vi "Intake Arm Controller.vi"(8 "error in":errorcluster) -> ()   [LabVIEW 2020]
doc: "This VI executes continuously carrying out the current operation and responding to updates or new operations. It will often contain the timing or control code that is difficult to place directly in TeleOp. This VI generally opens all sensors and motors and isolates the rest of the robot code from knowing how the operations are carried out."
uses:
  <vilib>/Rock Robotics/WPI/Framework/Completion Status.ctl
  Intake Arm Setpoints.ctl
  Intake Arm Operations.ctl
  <vilib>/Rock Robotics/WPI/Solenoid/WPI_SolenoidValue.ctl
  <vilib>/Rock Robotics/WPI/Solenoid/WPI_SolenoidChannel.ctl
  <vilib>/Rock Robotics/WPI/SafetyOutput/WPI_SafetyOutputConfigMenu.ctl
  <vilib>/Rock Robotics/WPI/Solenoid/WPI_SolenoidOpenDouble.vi
  <vilib>/Rock Robotics/WPI/Solenoid/WPI_SolenoidSetEnum.vi
  <vilib>/Rock Robotics/Network Tables/NT Write Number.vi
panel:
  in  "Interactive Values":T1
  out "Current\nCmd":string
  in  "Buttons":cluster{"Execute Cmd":bool, "Abort Cmd":bool}
  out "Command Timing":cluster{"Start Time (ms)":u32, "Iterations":i32}
  out "Status":T4
  # "Tip: It may be helpful to observe inputs and sensor values.\nYou may also want to display tuning or debugging controls."
  # "Interactive Command: You may fill in the settings for a command\nand schedule it with the Execute button. You can observe and abort\nany command while fine tuning the code for the controller."
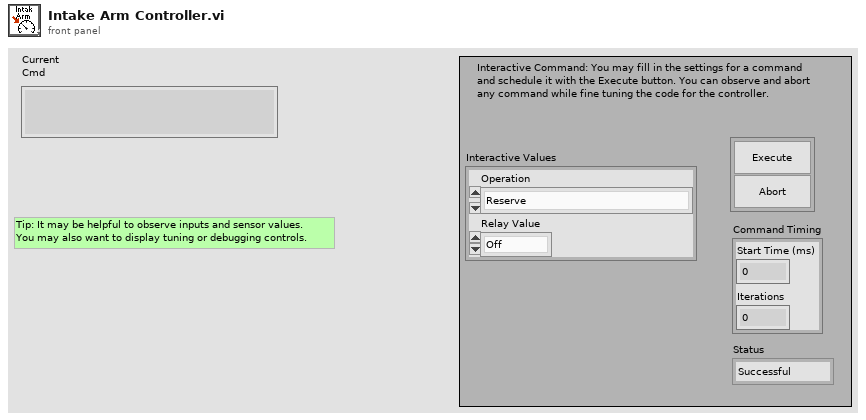
[diagram p1: front panel]
types:
  T1 = typedef "Intake Arm Setpoints.ctl" = cluster{"Operation":T2, "Relay Value":T3}
  T2 = typedef "Intake Arm Operations.ctl" = enum16{"Reserve", "Read Current", "Immediate", "Intake Arm Immediate", "Down", "Up"}
  T3 = typedef "WPI_SolenoidValue.ctl" = enum16{"Off", "On", "Forward", "Reverse"}
  T4 = typedef "Completion Status.ctl" = enum16{"Successful", "Aborted", "Incomplete"}
  T5 = typedef "WPI_SolenoidChannel.ctl" = enum8{"Solenoid 0", "Solenoid 1", "Solenoid 2", "Solenoid 3", "Solenoid 4", "Solenoid 5", "Solenoid 6", "Solenoid 7", "Solenoid 8", "Solenoid 9", "Solenoid 10", "Solenoid 11", "Solenoid 12", "Solenoid 13", "Solenoid 14", "Solenoid 15", "Invalid"}
  T6 = typedef "WPI_SafetyOutputConfigMenu.ctl" = enum16{"Enable", "Disable"}
  T7 = typedef "WPI_SolenoidDevRef.ctl" = cluster{"DevStatus":errorcluster, "Pneumatics Control Module":u8, "Forward Solenoid Channel":T5, "Reverse Solenoid Channel":T5}
  T8 = typedef "Command Status Info.ctl" = cluster{"Name":string, "Status":T4, "notifier out":T9}
  T9 = typedef "Completion Notifier.ctl" = refnum<notifier>
  T10 = cluster{"Current Command":T1, "Command Timing":cluster{"Start Time (ms)":u32, "Iterations":i32}, "Command Arguments":cluster{"Command Info":T8, "Description":string, "Default Command":T1, "queue out":refnum<queue>, "Subsystem Name":string}}
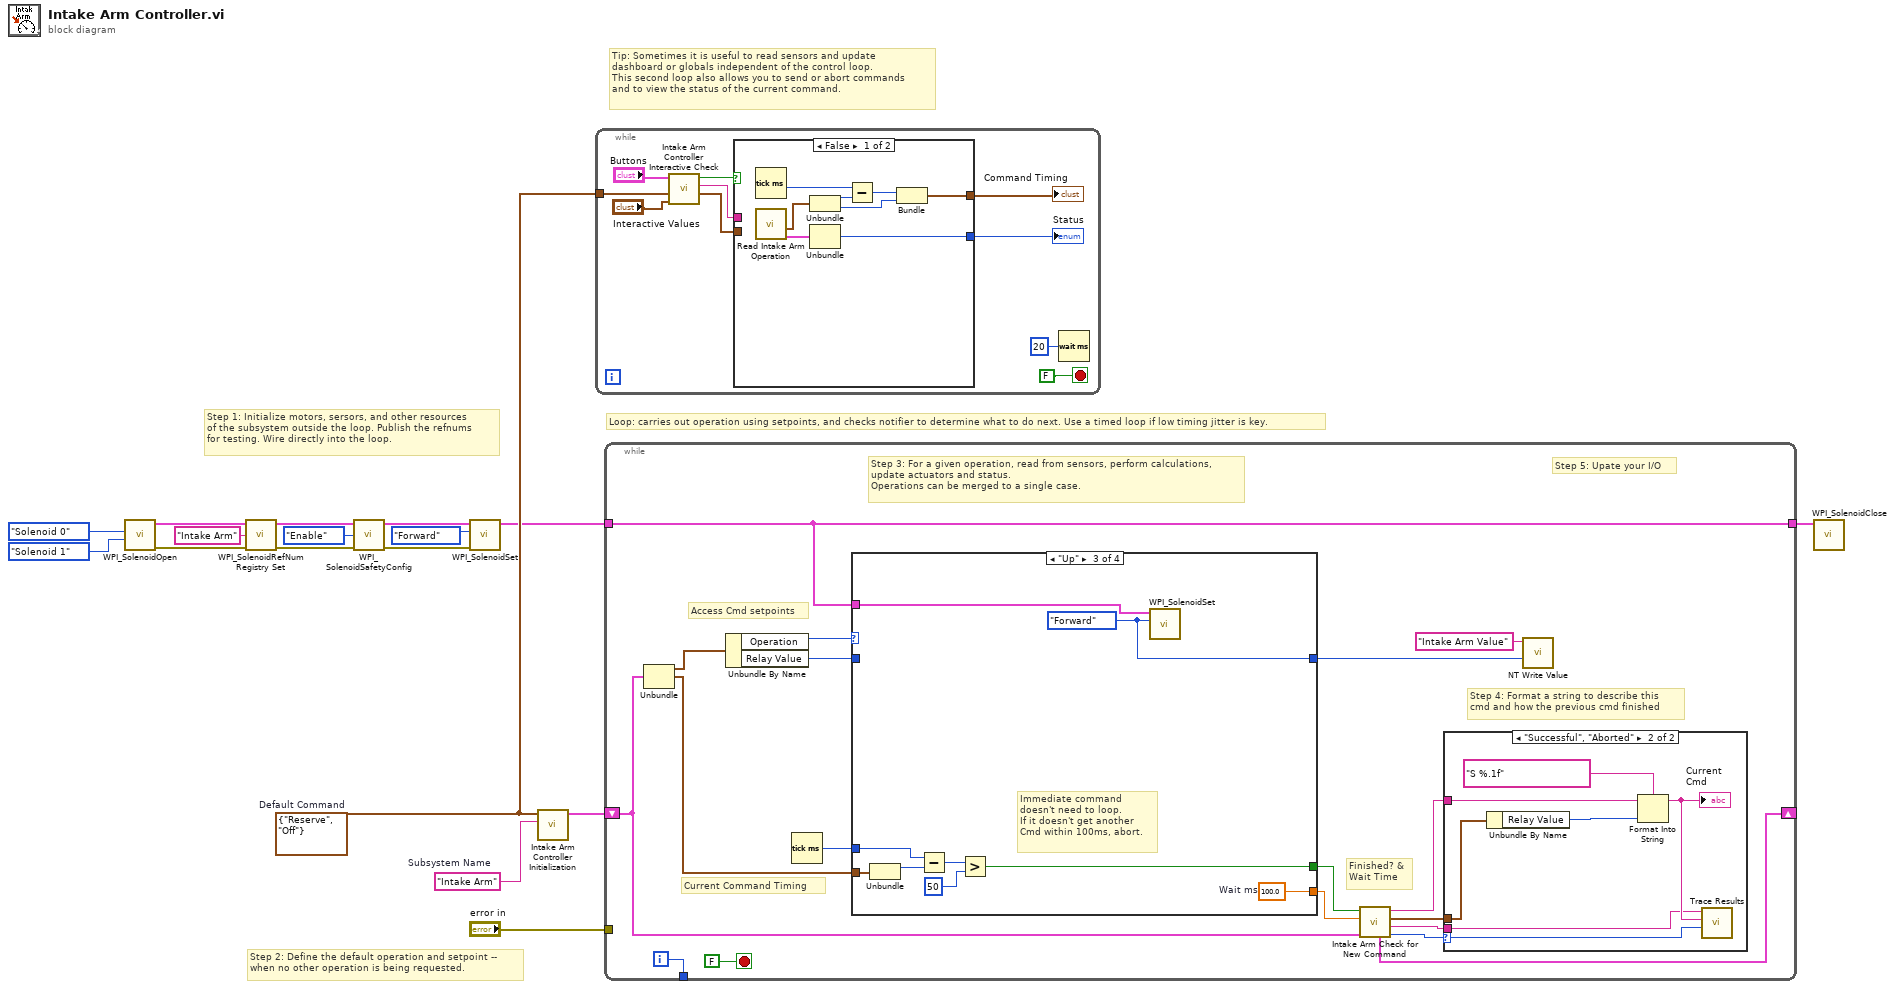
[diagram p0: block diagram]
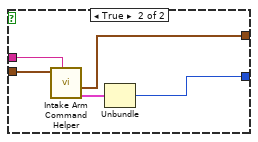
[diagram p2: hidden frame]
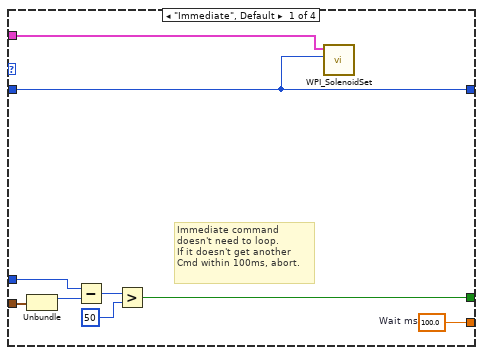
[diagram p4: hidden frame]
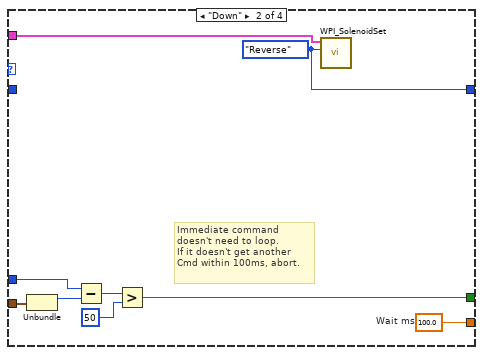
[diagram p5: hidden frame]
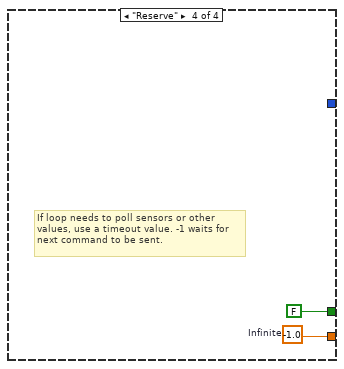
[diagram p6: hidden frame]
diagram:
  w14 = T1 {"Operation"=enum."Reserve", "Relay Value"=enum."Off"}  # Default Command
  w15 = "Intake Arm"  # Subsystem Name
  # "Tip: Sometimes it is useful to read sensors and update\ndashboard or globals independent of the control loop.\nThis second loop also allows you to send or abort commands\nand to view the status of the current command."
  # "Step 2: Define the default operation and setpoint --\nwhen no other operation is being requested."
  # "Step 1: Initialize motors, sersors, and other resources\nof the subsystem outside the loop. Publish the refnums\nfor testing. Wire directly into the loop."
  # "Loop: carries out operation using setpoints, and checks notifier to determine what to do next. Use a timed loop if low timing jitter is key."
  n1 = call-poly <vilib>:"WPI_SolenoidOpen.vi"("Reverse Solenoid Channel"=WPI_SolenoidChannel."Solenoid 1" ("Solenoid Channel"), "Forward Solenoid Channel"=WPI_SolenoidChannel."Solenoid 0" ("Solenoid Channel")) -> ("error out"=w10:errorcluster, "SolenoidDevRef"=w13:T7)  [unwired: 8 in]
  n2 = call <vilib>:"WPI_SolenoidRefNum Registry Set.vi"("error in (no error)"=w10, "refnum name"="Intake Arm", "SolenoidDevRef"=w13) -> ("error out"=w9:errorcluster, "SolenoidDevRef"=w12:T7)  [unwired: 7 in]
  n3 = call <vilib>:"WPI_SolenoidSafetyConfig.vi"("error in (no error)"=w9, "mode"=WPI_SafetyOutputConfigMenu."Enable", "SolenoidDevRef"=w12) -> ("error out"=w8:errorcluster, "SolenoidDevRef"=w11:T7)  [unwired: 7 in]
  n4 = call-poly <vilib>:"WPI_SolenoidSet.vi"("error in (no error)"=w8, "Value"=WPI_SolenoidValue."Forward", "SolenoidDevRef"=w11) -> ("SolenoidDevRef"=w2:T7)  [unwired: 7 in, 1 out]
  n5 = call "Intake Arm Controller Initialization.vi"("Subsystem Name"=w15, "Default Command"=w14) -> ("Current Command"=w16:T10)  [unwired: 9 in]
  n6 = while {
    tunnel: w14 -> [w24]
    stop <- FALSE stop-if-true
    n7 = call "Intake Arm Controller Interactive Check.vi"("Interactive Command in"="Interactive Values", "Default Command"=w24, "Buttons"="Buttons") -> ("Interactive Command out"=w21:T1, "Trace String"=w22:string, "Schedule"=w23:bool)  [unwired: 6 in]
    n8 = case shown="False" w23 {
      tunnel: [w35 w40] -> w20
      tunnel: w21 -> [_ w38]
      tunnel: [w31 w36] -> w19
      tunnel: w22 -> [_ w39]
      frame False {
        n9 = Tick Count (ms)() -> (millisecond timer value=w30:u32)
        n10 = call "Read Intake Arm Operation.vi"() -> ("Command Info"=w28:T8, "SubSystem Data"=w29:T1)  [unwired: 9 in, 1 out]
        n11 = Unbundle(w29) -> ("Operation"=w34:T2, "Relay Value"=w32:T3)
        n12 = Unbundle(w28) -> ("Status"=w35:T4)  [unwired: 2 out]
        n13 = Subtract(x=w30, y=w34) -> (x-y=w33:u32)
        n14 = Bundle(w33, "Relay Value"=w32) -> (w31:cluster{u32, "Relay Value":T3})  [unwired: 1 in]
      }
      frame True {
        n15 = call "Intake Arm Command Helper.vi"("Description"=w39, "SubSystem Data"=w38) -> ("Command Info Out"=w37:T8, "Command Timing"=w36:cluster{"Start Time (ms)":u32, "Iterations":i32})  [unwired: 7 in, 1 out]
        n16 = Unbundle(w37) -> ("Status"=w40:T4)  [unwired: 2 out]
      }
    }
    "Status" <- w20
    "Command Timing" <- w19
    n17 = Wait (ms)(milliseconds to wait=u32 20) -> ()  [unwired: 1 out]
  }
  n18 = while {
    shift-right: [w52] -> _
    shift-left: w16 -> [w45]
    tunnel: [w57] -> _
    tunnel: "error in" -> [_]
    tunnel: w2 -> [w41]
    tunnel: [w41] -> w1
    i -> [w57]
    stop <- FALSE stop-if-true
    # "Step 5: Upate your I/O"
    # "Step 4: Format a string to describe this\ncmd and how the previous cmd finished"
    # "Current Command Timing"
    # "Access Cmd setpoints"
    # "Finished? &\nWait Time"
    # "Step 3: For a given operation, read from sensors, perform calculations,\nupdate actuators and status.\nOperations can be merged to a single case."
    n19 = Unbundle(w45) -> ("Current Command"=w56:T1, "Command Timing"=w53:cluster{"Start Time (ms)":u32, "Iterations":i32})  [unwired: 1 out]
    n20 = Unbundle By Name(w56) -> ("Operation"=w55:T2, "Relay Value"=w44:T3)
    n21 = Tick Count (ms)() -> (millisecond timer value=w54:u32)
    n22 = case shown="\"Up\"" w55 {
      tunnel: [w74 w83 w92 w94] -> w50
      tunnel: [w68 w77 w86 FALSE ("ignore previous (F)")] -> w51
      tunnel: w53 -> [w70 w79 w88 _]
      tunnel: w54 -> [w69 w78 w87 _]
      tunnel: [w66 w75 w84 _] -> w43
      tunnel: w44 -> [w66 _ _ _]
      tunnel: w41 -> [w67 w76 w85 _]
      frame "Immediate", Default {
        w74 = 100.0  # Wait ms
        # "Immediate command\ndoesn't need to loop.\nIf it doesn't get another\nCmd within 100ms, abort."
        n23 = Unbundle(w70) -> ("Start Time (ms)"=w73:u32)  [unwired: 1 out]
        n24 = Subtract(x=w69, y=w73) -> (x-y=w72:u32)
        n25 = Greater?(x=w72, y=u8 50 ("Left Motor")) -> (0:w68:bool)
        n26 = call-poly <vilib>:"WPI_SolenoidSet.vi"("Value"=w66, "SolenoidDevRef"=w67) -> ()  [unwired: 8 in, 2 out]
      }
      frame "Down" {
        w75 = WPI_SolenoidValue."Reverse" ("Value")
        w83 = 100.0  # Wait ms
        # "Immediate command\ndoesn't need to loop.\nIf it doesn't get another\nCmd within 100ms, abort."
        n27 = Unbundle(w79) -> ("Start Time (ms)"=w82:u32)  [unwired: 1 out]
        n28 = Subtract(x=w78, y=w82) -> (x-y=w81:u32)
        n29 = Greater?(x=w81, y=u8 50 ("Left Motor")) -> (0:w77:bool)
        n30 = call-poly <vilib>:"WPI_SolenoidSet.vi"("Value"=w75, "SolenoidDevRef"=w76) -> ()  [unwired: 8 in, 2 out]
      }
      frame "Up" {
        w84 = WPI_SolenoidValue."Forward" ("Value")
        w92 = 100.0  # Wait ms
        # "Immediate command\ndoesn't need to loop.\nIf it doesn't get another\nCmd within 100ms, abort."
        n31 = Unbundle(w88) -> ("Start Time (ms)"=w91:u32)  [unwired: 1 out]
        n32 = Subtract(x=w87, y=w91) -> (x-y=w90:u32)
        n33 = Greater?(x=w90, y=u8 50 ("Left Motor")) -> (0:w86:bool)
        n34 = call-poly <vilib>:"WPI_SolenoidSet.vi"("Value"=w84, "SolenoidDevRef"=w85) -> ()  [unwired: 8 in, 2 out]
      }
      frame "Reserve" {
        w94 = -1.0  # Infinite
        # "If loop needs to poll sensors or other\nvalues, use a timeout value. -1 waits for\nnext command to be sent."
      }
    }
    n35 = call "Intake Arm Check for New Command.vi"("Current Command"=w45, "Wait time (ms)"=w50, "Finished?"=w51) -> ("Completion"=w46:T4, "Subsystem Name"=w47:string, "Current Command"=w48:T1, "Initial Trace String"=w49:string, "NextCommand"=w52:T10)  [unwired: 4 in]
    n36 = case shown="\"Successful\", \"Aborted\"" w46 {
      selector: w46 -> [_ w65]
      tunnel: w49 -> [_ w61]
      tunnel: w48 -> [_ w62]
      tunnel: w47 -> [_ w59]
      frame "Incomplete", Default {
        # "Continuing current command"
      }
      frame "Successful", "Aborted" {
        # "Report and setup for next command"
        n37 = Unbundle By Name(w62) -> ("Relay Value"=w64:T3)
        n38 = Format Into String(format string="S %.1f", initial string=w61, w64) -> (resulting string=w60:string)  [unwired: 1 in, 1 out]
        "Current\nCmd" <- w60
        n39 = call <vilib>:"Trace Results.vi"("Status of previous command"=w65, "Description"=w60, "Subsystem"=w59) -> ()  [unwired: 9 in]
      }
    }
    n40 = call-poly <vilib>:"NT Write Value.vi"("Numeric"=w43, "Name"="Intake Arm Value") -> ()  [unwired: 9 in, 1 out]
  }
  n41 = call <vilib>:"WPI_SolenoidClose.vi"("SolenoidDevRef"=w1) -> ()  [unwired: 10 in, 1 out]
